vi "Get Geometric Mean Longitude.vi"(11 "Julian Century":dbl) -> (3 "Geometric Mean Longitude":dbl)   [LabVIEW 2013, in "Solar Calculations.lvlib"]
doc: "Calculate the geometric mean longitude of the sun freed from aberation."
uses:
  Solar Calculations.lvlib
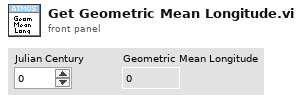
[diagram p1: front panel]
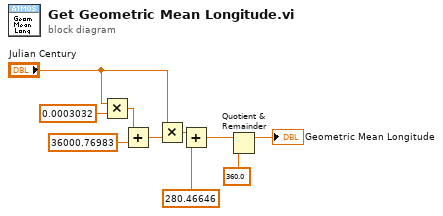
[diagram p0: block diagram]
diagram:
  n1 = Multiply(x="Julian Century", y=0.0003032) -> (x*y=w3:dbl)
  n2 = Add(x=w3, y=36000.76983) -> (x+y=w5:dbl)
  n3 = Multiply(x="Julian Century", y=w5) -> (x*y=w7:dbl)
  n4 = Add(x=w7, y=280.46646) -> (x+y=w8:dbl)
  n5 = Quotient & Remainder(x=w8, y=360.0) -> (x-y*floor(x/y)=→"Geometric Mean Longitude":dbl)  [unwired: 1 out]
